vi "example 7 - grand child.vi"() -> ()   [LabVIEW 2020]
panel:
  in  "Cluster":T1
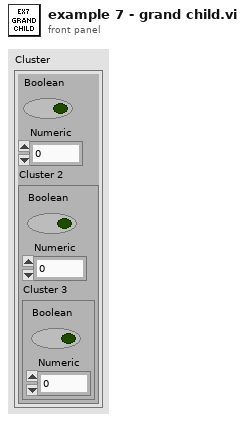
[diagram p1: front panel]
types:
  T1 = cluster{"Boolean":bool, "Numeric":dbl, "Cluster 2":cluster{"Boolean":bool, "Numeric":dbl, "Cluster 3":cluster{"Boolean":bool, "Numeric":dbl}}}
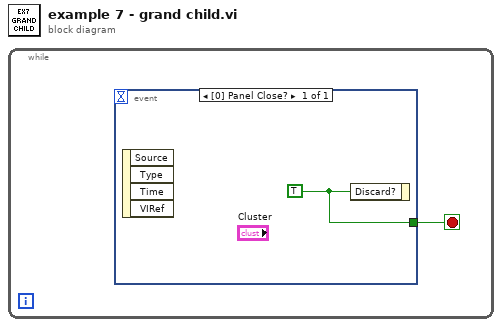
[diagram p0: block diagram]
diagram:
  n1 = while {
    stop <- w1 stop-if-true
    n2 = event shown="[0] Panel Close?" {
      selector: _ -> [_]
      dyn-events: _ -> [_]
      timeout: _ -> [_]
      tunnel: [w2] -> w1
      event Panel Close? {
        w2 = TRUE
        n3 = event-data() -> ()  [unwired: 1 in, 4 out]
        n4 = event-data("Discard?"=w2) -> ()  [unwired: 1 in, 1 out]
      }
    }
  }
